vi "RegisterTrendPoints.vi"(8 "error in (no error)":errorcluster, 10 "register trend":T1, 11 "registry in":variant) -> (0 "error out":errorcluster, 3 "registry out":variant)   [LabVIEW 2017, in "McsaDataEventCreator.lvlib"]
uses:
  <vilib>/addons/InsightCM/Devices/Shared/Mcsa/McsaDataEventCreator/McsaDataEventCreator.lvlib
  <vilib>/addons/InsightCM/Devices/Shared/Common/DataEventCreator/controls/RegisterTrendPoints.ctl
  <vilib>/addons/InsightCM/Devices/Shared/Common/DataEventCreator/controls/Registry_Trend.ctl
  <vilib>/addons/InsightCM/Devices/Shared/Mcsa/McsaDataEventCreator/controls/DataGroupRegistry.ctl
  <vilib>/addons/InsightCM/Devices/Shared/Mcsa/McsaDataEventCreator/controls/Registry_DataSet.ctl
  <vilib>/addons/InsightCM/Devices/Shared/Mcsa/McsaDataEventCreator/controls/DataSetType.ctl
  <vilib>/addons/InsightCM/Devices/Shared/Common/DataEventCreator/DataEventCreator.lvlib
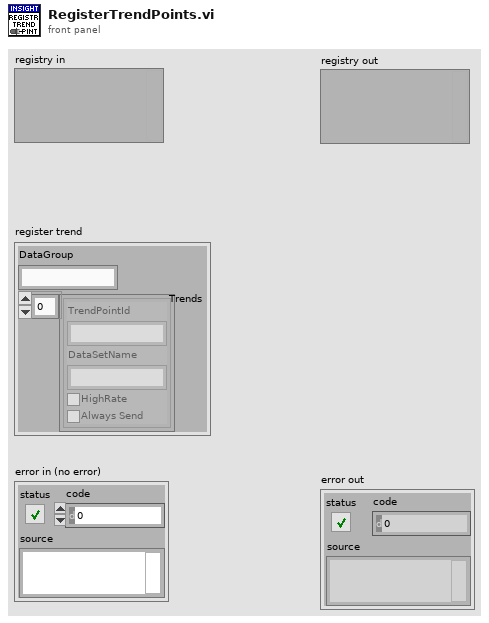
[diagram p1: front panel]
types:
  T1 = typedef "DataEventCreator.lvlib/RegisterTrendPoints.ctl" = cluster{"DataGroup":string, "Trends":T2[]}
  T2 = typedef "DataEventCreator.lvlib/Registry_Trend.ctl" = cluster{"TrendPointId":string, "DataSetName":string, "HighRate":bool, "Always Send":bool}
  T3 = typedef "McsaDataEventCreator.lvlib/DataGroupRegistry.ctl" = cluster{"AssetNodeMap":variant, "DataSets":T4[], "Trends":T2[]}
  T4 = typedef "McsaDataEventCreator.lvlib/Registry_DataSet.ctl" = cluster{"ChannelName":string, "DataSetType":T5, "DoNotWriteToDB":bool, "ParentName":string}
  T5 = typedef "McsaDataEventCreator.lvlib/DataSetType.ctl" = enum16{"Waveform", "MCSAFFT", "TorqueWFM"}
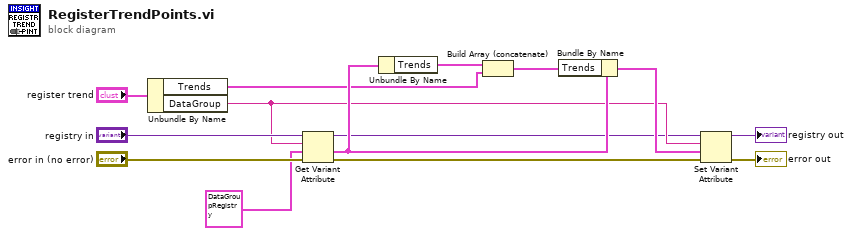
[diagram p0: block diagram]
diagram:
  n1 = Unbundle By Name("register trend") -> ("Trends"=w1:T2[], "DataGroup"=w8:string)
  n2 = Get Variant Attribute(Variant="registry in", name=w8, default value (empty Variant)=T3 {"AssetNodeMap"=variant, "DataSets"=[], "Trends"=[]} ("Data Group Registry"), error in="error in (no error)") -> (duplicate Variant=w4:variant, value=w11:T3, error out=w5:errorcluster)  [unwired: 1 out]
  n3 = Unbundle By Name(w11) -> ("Trends"=w14:T2[])
  n4 = Build Array (concatenate)(w14, w1) -> (w10:T2[])
  n5 = Bundle By Name(cluster=w11, "Trends"=w10) -> (w9:T3)
  n6 = Set Variant Attribute(Variant=w4, name=w8, value=w9, error in=w5) -> (Variant out=→"registry out":variant, error out=→"error out":errorcluster)  [unwired: 1 out]
